vi "Nicmos_LogTemperature.vi"() -> ()   [LabVIEW 2009]
uses:
  <vilib>/Utility/file.llb/Read From Spreadsheet File (DBL).vi
  <vilib>/Utility/file.llb/Write To Spreadsheet File (DBL).vi
panel:
  out "Temperature Graph":cluster{timestamp[], "all rows":dbl[]}[](graph)
  in  "stop":bool
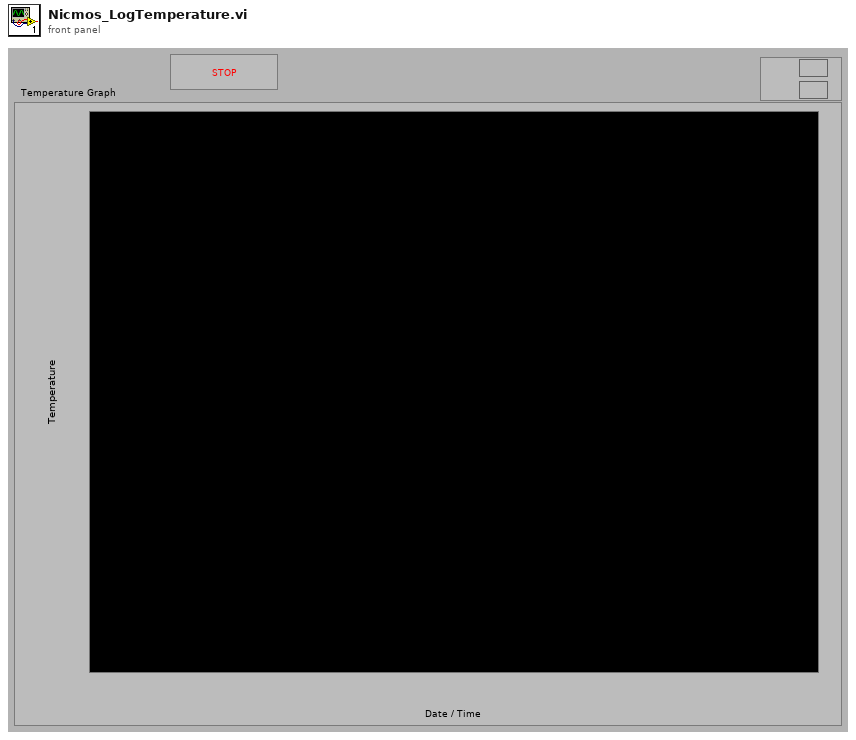
[diagram p1: front panel]
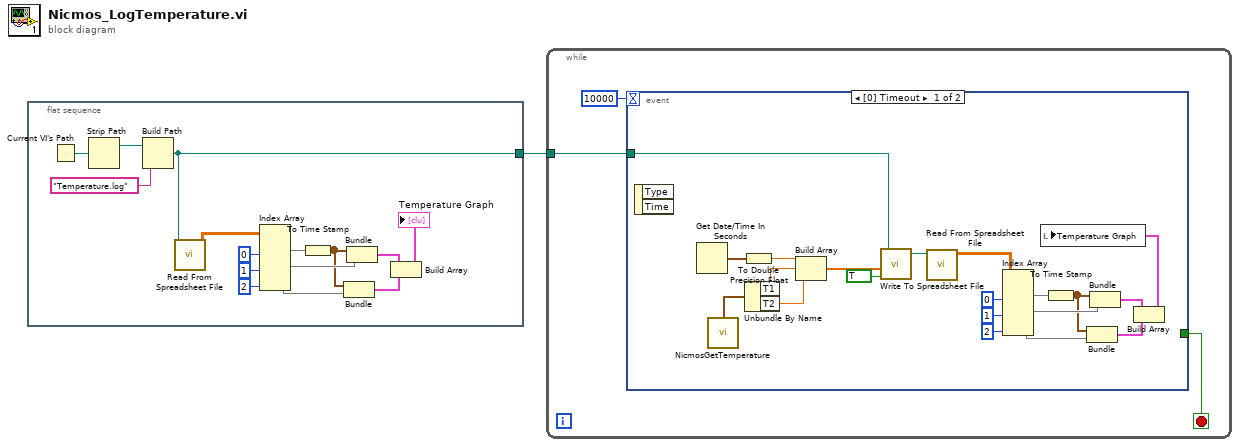
[diagram p0: block diagram]
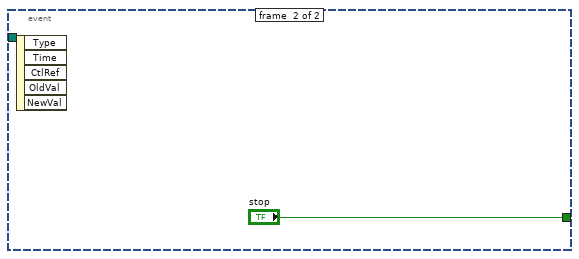
[diagram p2: hidden frame]
diagram:
  n1 = flat-sequence {
    tunnel: [w13] -> w1
    frame #0 {
      n2 = Current VI's Path() -> (path=w14:path)
      n3 = Strip Path(path=w14) -> (stripped path=w15:path)  [unwired: 1 out]
      n4 = Build Path(base path=w15, name or relative path="Temperature.log") -> (appended path=w13:path)
      n5 = call-poly <vilib>:"Read From Spreadsheet File.vi"("file path (dialog if empty)"=w13) -> ("all rows"=w12:dbl[][])  [unwired: 6 in, 4 out]
      n6 = Index Array(array=w12, index (col) #1=0 ("disabled index (col)"), index (col) #2=1 ("index (col)"), index (col) #3=2 ("index (col)")) -> (element #1=w8:dbl[], element #2=w7:dbl[], element #3=w6:dbl[])  [unwired: 3 in]
      n7 = To Time Stamp(1:w8) -> (0:w5:timestamp[])
      n8 = Bundle(w5, "all rows"=w6) -> (w3:cluster{timestamp[], "all rows":dbl[]})  [unwired: 1 in]
      n9 = Bundle(w5, "all rows"=w7) -> (w4:cluster{timestamp[], "all rows":dbl[]})  [unwired: 1 in]
      n10 = Build Array(w4, w3) -> (→"Temperature Graph":cluster{timestamp[], "all rows":dbl[]}[])
    }
  }
  n11 = while {
    tunnel: w1 -> [w17]
    stop <- w18 stop-if-true
    n12 = event shown="[0] Timeout" {
      selector: _ -> [_ _]
      dyn-events: _ -> [_ _]
      timeout: 10000 -> [_ _]
      tunnel: [_ "stop"] -> w18
      tunnel: w17 -> [w32 _]
      event #0 {
        n13 = event-data() -> ()  [unwired: 1 in, 2 out]
        n14 = Get Date/Time In Seconds() -> (seconds since 1Jan1904=w37:timestamp)
        n15 = call "NicmosGetTemperature.vi"() -> ("Temperature graph"=w38:cluster{"T1":dbl, "T2":dbl})  [unwired: 8 in, 1 out]
        n16 = To Double Precision Float(number=w37) -> (double precision float=w36:dbl)
        n17 = Unbundle By Name(w38) -> ("T1"=w35:dbl, "T2"=w34:dbl)
        n18 = Build Array(w36, w35, w34) -> (w33:dbl[])
        n19 = call-poly <vilib>:"Write To Spreadsheet File.vi"("append to file? (new file:F)"=TRUE, "1D data"=w33, "file path (dialog if empty)"=w32) -> ("new file path (Not A Path if cancelled)"=w22:path)  [unwired: 5 in]
        n20 = call-poly <vilib>:"Read From Spreadsheet File.vi"("file path (dialog if empty)"=w22) -> ("all rows"=w21:dbl[][])  [unwired: 6 in, 4 out]
        n21 = Index Array(array=w21, index (col) #1=0 ("disabled index (col)"), index (col) #2=1 ("index (col)"), index (col) #3=2 ("index (col)")) -> (element #1=w28:dbl[], element #2=w27:dbl[], element #3=w26:dbl[])  [unwired: 3 in]
        n22 = To Time Stamp(1:w28) -> (0:w25:timestamp[])
        n23 = Bundle(w25, "all rows"=w26) -> (w23:cluster{timestamp[], "all rows":dbl[]})  [unwired: 1 in]
        n24 = Bundle(w25, "all rows"=w27) -> (w24:cluster{timestamp[], "all rows":dbl[]})  [unwired: 1 in]
        n25 = Build Array(w24, w23) -> (w20:cluster{timestamp[], "all rows":dbl[]}[])
        n26 = local write "Temperature Graph"(w20) -> ()
      }
      event #1 {
        n27 = event-data() -> ()  [unwired: 1 in, 5 out]
      }
    }
  }
